vi "communicate.vi"(0 "Communication in":refnum<class "Communication.lvclass">, 1 "grSIM replacement":cluster{"robots":T4[], "ball":T5}, 2 "replace active":bool, 5 "Game":refnum<class "Game.lvclass">, 7 "Com UDP":T3={"UDP GrSim TX"=TRUE, "Address:"="127.0.0.1", "Port:"=20011}, 9 "Com Serial":T2, 11 "error in (no error)":errorcluster, 12 "Com SOS":T1={"UDP SOS TX "=FALSE, "SOS Port: 2"=10025, "SOS Port: "=10021, "SOS Address:"="192.168.0.101"}) -> (4 "Communication out":refnum<class "Communication.lvclass">, 6 "Comm TX FPS":dbl, 10 "AllyRef":refnum<class "Ally.lvclass">, 15 "error out":errorcluster)   [LabVIEW 2018, in "Communication.lvclass"]
uses:
  Communication.lvclass
  Paths/grSim Packet Command UDP Test Folder/grSim/grSim RobotReplacement.ctl
  Paths/grSim Packet Command UDP Test Folder/grSim/grSim_BallReplacement.ctl
  Vision_class/Old vision/SSL Detection Frame Simple Estimator Cameras VelCmd Folder/Core/AI Input.ctl
  Vision_class/Old vision/Controls/AI Robot.ctl
  Vision_class/Old vision/Controls/Functions Enum.ctl
  Vision_class/Old vision/Controls/AttackerStates.ctl
  Vision_class/Old vision/Controls/PathDests.ctl
  Vision_class/Old vision/Controls/PathDest.ctl
  Vision_class/Old vision/SSL Detection Frame Simple Estimator Cameras VelCmd Folder/Core/AI Ball.ctl
  Vision_class/Old vision/SSL Detection Frame Simple Estimator Cameras VelCmd Folder/Core/Field Size.ctl
  Vision_class/Old vision/SSL Detection Frame Simple Estimator Cameras VelCmd Folder/Core/AI Judge.ctl
  Paths/MessageAI_State Folder/Intel/Command Enum.ctl
  Vision_class/Old vision/SSL Detection Frame Simple Estimator Cameras VelCmd Folder/Util/Events/Events.ctl
  Game_class/Game.lvclass
  Controls/ComUDP.ctl
  Controls/ComSerial.ctl
  Controls/ComSOS.ctl
  Ally_class/Ally.lvclass
panel:
  in  "IA States":T6={"our_robots"=[], "enemy_robots"=[], "balls"=[], "geometry"={"line_width"=0, "field_length"=0, "field_width"=0, "boundary_width"=0, "referee_width"=0, "goal_width"=0, "goal_depth"=0, "goal_wall_width"=0, "center_circle_radius"=0, "defense_radius"=0, "defense_stretch"=0, "free_kick_from_defense_dist"=0, "penalty_spot_from_field_line_dist"=0, "penalty_line_from_spot_dist"=0}, "IA Judge"={"stage"="", "command"="", "our_goalie_id"=0.0, "enemy_goalie_id"=0.0, "command enum"=enum."Halt", "Time"=enum."Azul"}, "Received Timestamp"=timestamp(0 s since 1904-01-01), "Events"={"Touch"=FALSE, "Ball out"=FALSE, "id touch"=0.0, "Ball out of \nVision"=FALSE, "Ball inside \nGoalie area"=FALSE, "Robot not responding"=FALSE, "Robots responding status"=[1.0, 1.0, 1.0, 1.0, 1.0, 1.0], "Enemy Ball \nPossession"=FALSE, "Pass State"=FALSE, "id end of pass"=0.0, "Kick"=FALSE, "Id ini Possession"=0.0, "Ball Possesion"=FALSE, "Id Possesion"=0.0, "Direct Kick"=FALSE, "2nd Strk Ativo"=FALSE}}
  out "grSim":cluster{"robots":T4[], "ball":T5}
  out "Total Delay":dbl format="%#.5g"
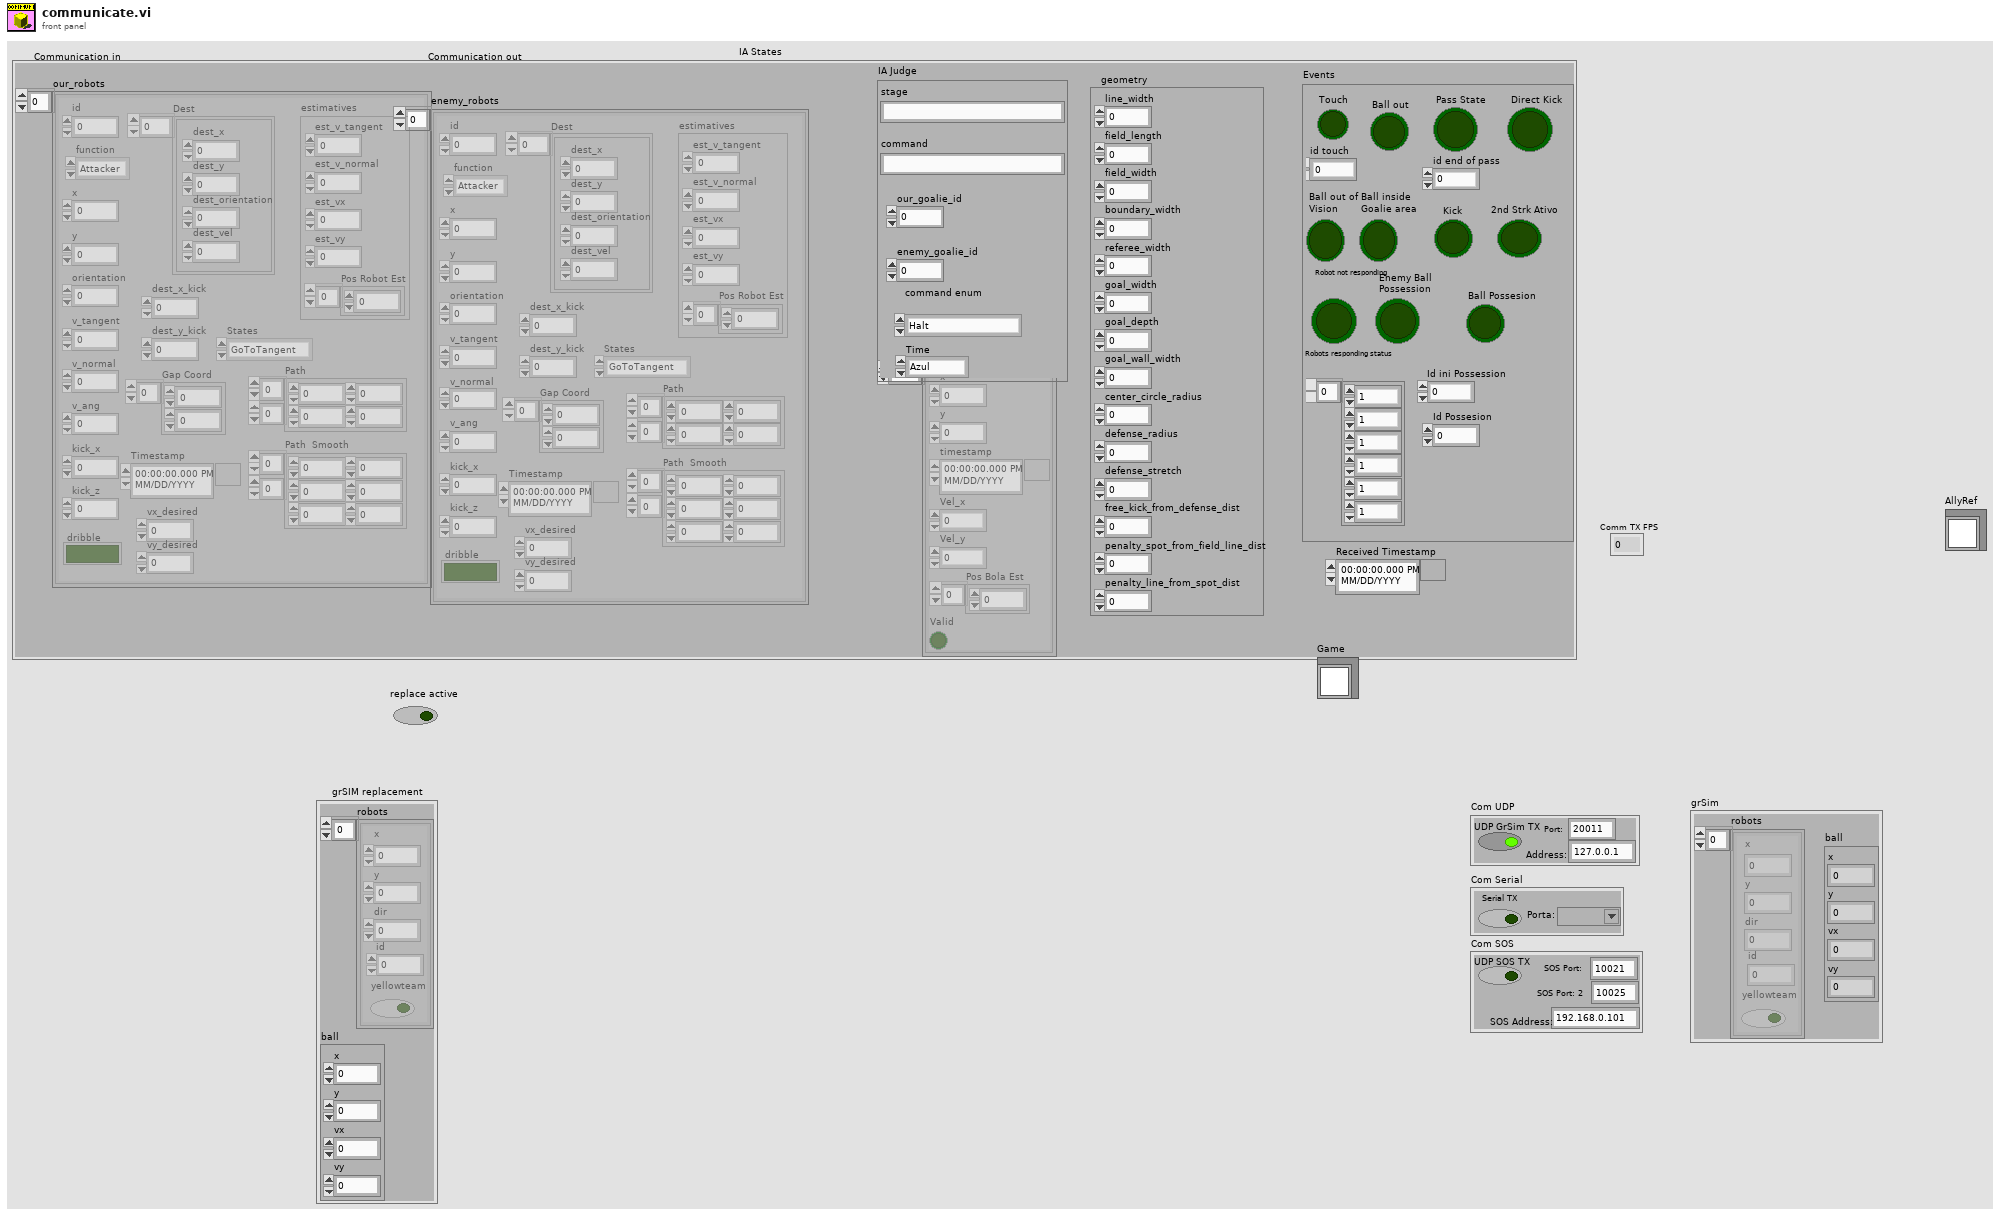
[diagram p1: front panel]
types:
  T1 = typedef "ComSOS.ctl" = cluster{"UDP SOS TX ":bool, "SOS Port: 2":u16, "SOS Port: ":u16, "SOS Address:":string}
  T2 = typedef "ComSerial.ctl" = cluster{"Serial TX":bool, "Porta:":refnum<visa-resource-name>}
  T3 = typedef "ComUDP.ctl" = cluster{"UDP GrSim TX":bool, "Address:":string, "Port:":u16}
  T4 = typedef "grSim RobotReplacement.ctl" = cluster{"x":dbl, "y":dbl, "dir":dbl, "yellowteam":bool, "id":u32}
  T5 = typedef "grSim_BallReplacement.ctl" = cluster{"x":dbl, "y":dbl, "vx":dbl, "vy":dbl}
  T6 = typedef "AI Input.ctl" = cluster{"our_robots":T7[], "enemy_robots":T7[], "balls":T12[], "geometry":T13, "IA Judge":T14, "Received Timestamp":timestamp, "Events":T16}
  T7 = typedef "AI Robot.ctl" = cluster{"id":u32, "function":T8, "x":dbl, "y":dbl, "orientation":dbl, "v_tangent":dbl, "v_normal":dbl, "v_ang":dbl, "kick_x":dbl, "kick_z":dbl, "dribble":bool, "Timestamp":timestamp, "estimatives":cluster{"est_v_tangent":dbl, "est_v_normal":dbl, "est_vx":dbl, "est_vy":dbl, "Pos Robot Est":dbl[]}, "dest_x_kick":dbl, "dest_y_kick":dbl, "Gap Coord":dbl[], "States":T9, "Path ":dbl[][], "Path  Smooth":dbl[][], "Dest":T10, "vx_desired":dbl, "vy_desired":dbl}
  T8 = typedef "Functions Enum.ctl" = enum16{"2nd Striker", "Attacker", "Goalie", "Defender", "Striker", "Goto 0", "Dummy", "Kicker", "ZigZag 0", "ZigZag 1", "ZigZag 2", "ZigZag 3", "ZigZag 4", "ZigZag 5", "ZigZag 6", "ZigZag 7", "ZigZag 8", ""}
  T9 = typedef "AttackerStates.ctl" = enum16{"Pass", "GoToTangent", "BallGetting", "GoToKick", ""}
  T10 = typedef "PathDests.ctl" = T11[]
  T11 = typedef "PathDest.ctl" = cluster{"dest_x":dbl, "dest_y":dbl, "dest_orientation":dbl, "dest_vel":dbl}
  T12 = typedef "AI Ball.ctl" = cluster{"x":dbl, "y":dbl, "timestamp":timestamp, "Vel_x":dbl, "Vel_y":dbl, "Pos Bola Est":dbl[], "Valid":bool}
  T13 = typedef "Field Size.ctl" = cluster{"line_width":u32, "field_length":u32, "field_width":u32, "boundary_width":u32, "referee_width":u32, "goal_width":u32, "goal_depth":u32, "goal_wall_width":u32, "center_circle_radius":u32, "defense_radius":u32, "defense_stretch":u32, "free_kick_from_defense_dist":u32, "penalty_spot_from_field_line_dist":u32, "penalty_line_from_spot_dist":u32}
  T14 = typedef "AI Judge.ctl" = cluster{"stage":string, "command":string, "our_goalie_id":dbl, "enemy_goalie_id":dbl, "command enum":T15, "Time":enum16{"Azul", "Amarelo"}}
  T15 = typedef "Command Enum.ctl" = enum16{"Halt", "Stop", "Force Start", "PKA Normal Start", "Prepare Kickoff Ally", "PKE Normal Start", "Prepare Kickoff Enemy", "Prepare Penalty Ally", "PPA Normal Start", "Prepare Penalty Enemy", "PPE Normal Start", "Direct Free Enemy", "Direct Free Ally", "Indirect Free Enemy", "Indirect Free Ally", "Timeout Enemy", "Timeout Ally", "Goal Enemy", "Goal Ally", "Ball Placement Enemy", "Ball Placement Ally", "Normal Half Time", "Extra Time Break", "Extra Half Time", "None", "Post Game"}
  T16 = typedef "Events.ctl" = cluster{"Touch":bool, "Ball out":bool, "id touch":dbl, "Ball out of \nVision":bool, "Ball inside \nGoalie area":bool, "Robot not responding":bool, "Robots responding status":dbl[], "Enemy Ball \nPossession":bool, "Pass State":bool, "id end of pass":dbl, "Kick":bool, "Id ini Possession":dbl, "Ball Possesion":bool, "Id Possesion":dbl, "Direct Kick":bool, "2nd Strk Ativo":bool}
  T17 = typedef "grSim Robot Command.ctl" = cluster{"id":u32, "kickspeedx":sgl, "kickspeedz":sgl, "veltangent":sgl, "velnormal":sgl, "velangular":sgl, "spinner":bool, "wheelspeed":bool, "wheel1":sgl, "wheel2":sgl, "wheel3":sgl, "wheel4":sgl}
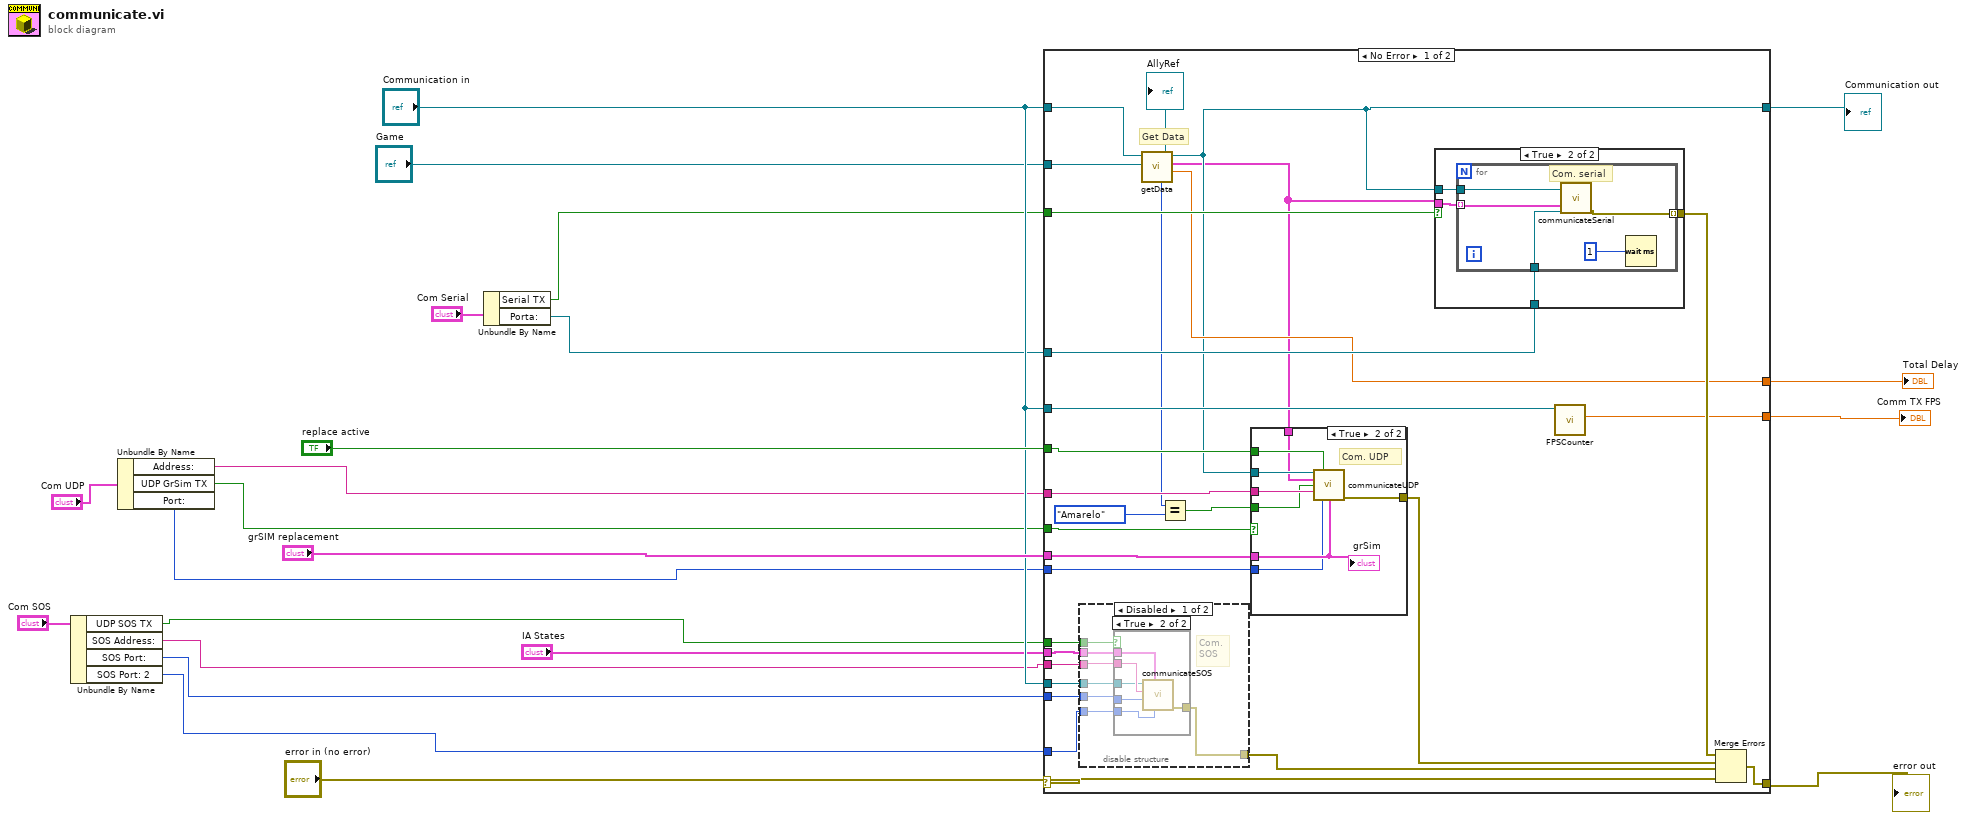
[diagram p0: block diagram]
diagram:
  n1 = Unbundle By Name("Com SOS") -> ("UDP SOS TX"=w7:bool, "SOS Address:"=w6:string, "SOS Port:"=w5:u16, "SOS Port: 2"=w4:u16)
  n2 = Unbundle By Name("Com UDP") -> ("Address:"=w11:string, "UDP GrSim TX"=w10:bool, "Port:"=w9:u16)
  n3 = Unbundle By Name("Com Serial") -> ("Serial TX"=w1:bool, "Porta:"=w2:refnum<visa-resource-name>)
  n4 = case shown="No Error" "error in (no error)" {
    selector: "error in (no error)" -> [w37 w83]
    tunnel: [w38 w83] -> w18
    tunnel: [w27 w82] -> w21
    tunnel: "Communication in" -> [w28 w82]
    tunnel: "IA States" -> [w48 _]
    tunnel: "grSIM replacement" -> [w50 _]
    tunnel: "replace active" -> [w45 _]
    tunnel: w10 -> [w49 _]
    tunnel: w9 -> [w47 _]
    tunnel: w11 -> [w46 _]
    tunnel: w7 -> [w44 _]
    tunnel: w5 -> [w43 _]
    tunnel: w4 -> [w42 _]
    tunnel: w6 -> [w41 _]
    tunnel: w1 -> [w40 _]
    tunnel: w2 -> [w39 _]
    tunnel: "Communication in" -> [w34 _]
    tunnel: "Communication in" -> [w33 _]
    tunnel: [w31 _] -> w16
    tunnel: [w29 _] -> w15
    tunnel: "Game" -> [w25 _]
    frame No Error {
      # "Get Data"
      n5 = disable-structure shown="Disabled" {
        disable-tunnel: w48 -> [w58 _]
        disable-tunnel: w44 -> [w57 _]
        disable-tunnel: w43 -> [w56 _]
        disable-tunnel: w42 -> [w55 _]
        disable-tunnel: w41 -> [w54 _]
        disable-tunnel: [w53 _] -> w36
        disable-tunnel: w34 -> [w52 _]
        frame Disabled {
          # "Com.\nSOS"
          n6 = case shown="True" w57 {
            tunnel: w58 -> [_ w64]
            tunnel: w56 -> [_ w62]
            tunnel: w55 -> [_ w61]
            tunnel: w54 -> [_ w63]
            tunnel: [_ w60] -> w53
            tunnel: w52 -> [_ w59]
            frame False {
            }
            frame True {
              n7 = call-dynamic "communicateSOS.vi"("SOS Port: 2"=w61, "AI State"=w64, "SOS Port:"=w62, "SOS Address:"=w63, "Communication in"=w59) -> ("error out"=w60:errorcluster)  [unwired: 5 in, 1 out]
            }
          }
        }
        frame Enabled {
        }
      }
      n8 = call-dynamic "getData.vi"("Game"=w25, "Communication in"=w28) -> ("Total Delay"=w29:dbl, "Robot Data"=w24:T17[], "Communication out"=w27:refnum<class "Communication.lvclass">, "Team Color"=w26:enum16{"Azul", "Amarelo"}, "AllyRef"=→"AllyRef":refnum<class "Ally.lvclass">)  [unwired: 4 in, 1 out]
      n9 = Equal?(x=w26, y=enum16{"Azul", "Amarelo"}."Amarelo") -> (x = y?=w51:bool)
      n10 = case shown="True" w49 {
        tunnel: w51 -> [_ w77]
        tunnel: w45 -> [_ w76]
        tunnel: w50 -> [_ w81]
        tunnel: w47 -> [_ w80]
        tunnel: w46 -> [_ w78]
        tunnel: [_ w79] -> w35
        tunnel: w27 -> [_ w75]
        tunnel: w24 -> [_ w74]
        frame False {
        }
        frame True {
          # "Com. UDP"
          n11 = call-dynamic "communicateUDP.vi"("Communication in"=w75, "Replace Now"=w76, "Robots"=w74, "isMyTeamYellow"=w77, "Address:"=w78, "Port:"=w80, "grSim replacement"=w81) -> ("error out"=w79:errorcluster)  [unwired: 7 in, 1 out]
          "grSim" <- w81
        }
      }
      n12 = case shown="True" w40 {
        tunnel: w24 -> [_ w68]
        tunnel: w39 -> [_ w67]
        tunnel: [_ w66] -> w32
        tunnel: w27 -> [_ w65]
        frame False {
        }
        frame True {
          n13 = for {
            tunnel: w68 -> [w72] mode=indexing
            tunnel: w67 -> [w71]
            tunnel: [w70] -> w66 mode=indexing
            tunnel: w65 -> [w69]
            # "Com. serial"
            n14 = call-dynamic "communicateSerial.vi"("Porta:"=w71, "Robots"=w72, "Communication in"=w69) -> ("error out"=w70:errorcluster)  [unwired: 7 in, 1 out]
            n15 = Wait (ms)(milliseconds to wait=u32 1) -> ()  [unwired: 1 out]
          }
        }
      }
      n16 = call-dynamic "FPSCounter.vi"("Communication in"=w33) -> ("Comm TX FPS"=w31:dbl)  [unwired: 8 in, 2 out]
      n17 = Merge Errors(w32, w35, w36, w37) -> (w38:errorcluster)
    }
    frame Error {
    }
  }
  "error out" <- w18
  "Communication out" <- w21
  "Comm TX FPS" <- w16
  "Total Delay" <- w15
